vi "Close.vi"(8 "error in (no error)":errorcluster, 9 "timeout ms (5000)":i32=5000, 11 "WebSocket in":refnum<class "WebSocket.lvclass">) -> (0 "error out":errorcluster, 3 "TCP Connection out":refnum<k5>)   [LabVIEW 2021, in "WebSockets.lvlib"]
doc: "**Deprecated - please use the new WebSocket.lvclass VIs instead. VI is retained for backwards compatibility.**\n\nSends the shutdown opcode to the TCP socket. This VI will run even if an upstream error has occurred.\n\nNote: This does not close the TCP connection as you may want to wait for the shutdown opcode to be received from the client.\nWebSockets 2.0.1.40\nSam Sharp - MediaMongrels Ltd\nCopyright (c) 2019, MediaMongrels Ltd"
uses:
  WebSockets.lvlib
  WebSocket/WebSocket.lvclass
  Sockets/VISA TCP Socket/VISA TCP.lvclass
  WebSocket/WebSocket.lvclass/WebSocket.ctl
  Sockets/VISA TCP Socket/VISA TCP.lvclass/VISA TCP.ctl
  WebSocket/Read Socket.vi
  Sockets/VISA TCP Socket/Read TCP Refnum.vi
  Sockets/Socket/Socket.lvclass
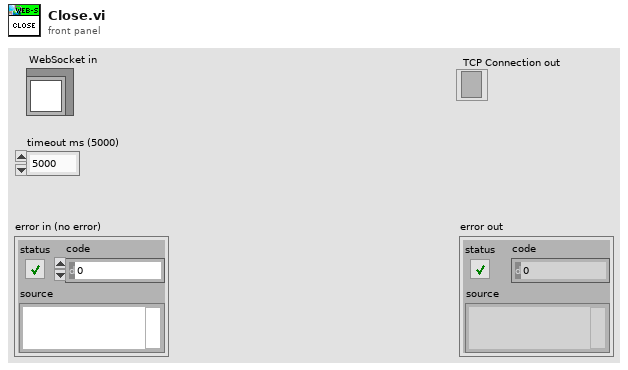
[diagram p1: front panel]
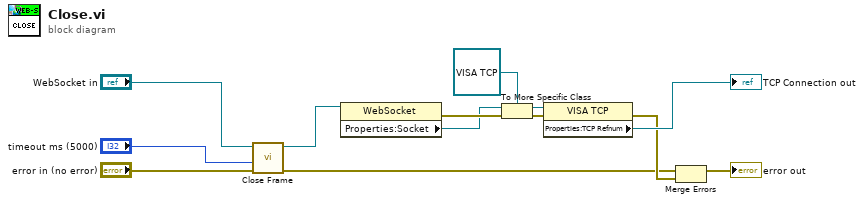
[diagram p0: block diagram]
diagram:
  n1 = call-dynamic "Close Frame.vi"("error in (no error)"="error in (no error)", "timeout ms (5000)"="timeout ms (5000)", "WebSockets in"="WebSocket in") -> ("error out"=w2:errorcluster, "WebSockets out"=w9:refnum<class "WebSocket.lvclass">)  [unwired: 7 in]
  n2 = property class="WebSocket"(reference=w9) -> (error out=w8:errorcluster, "Properties:Socket"=w7:refnum<class "Socket.lvclass">)  [unwired: 1 in, 1 out]
  n3 = To More Specific Class(target class=refnum<class "VISA TCP.lvclass"> refnum ("Socket.lvlib:VISA TCP"), reference=w7, error in=w8) -> (specific class reference=w4:refnum<class "VISA TCP.lvclass">, error out=w5:errorcluster)
  n4 = property class="VISA TCP"(reference=w4, error in=w5) -> (error out=w3:errorcluster, "Properties:TCP Refnum"=→"TCP Connection out":refnum<k5>)  [unwired: 1 out]
  n5 = Merge Errors(w2, w3) -> (→"error out":errorcluster)
